vi "CombineHiLoBytes.vi"(1 "unsigned byte array":u8[](array[numeric])) -> (0 "Numeric":u16)   [LabVIEW 2017, in "Spectral Products CM110.lvlib"]
uses:
  Spectral Products CM110.lvlib
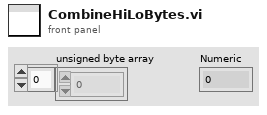
[diagram p1: front panel]
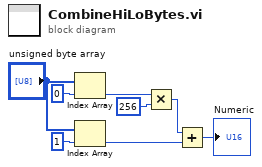
[diagram p0: block diagram]
diagram:
  n1 = Index Array(array="unsigned byte array", index=0) -> (element=w3:u8)
  n2 = Index Array(array="unsigned byte array", index=1) -> (element=w6:u8)
  n3 = Multiply(x=w3, y=u16 256) -> (x*y=w5:u16)
  n4 = Add(x=w5, y=w6) -> (x+y=→"Numeric":u16)
